vi "A320飞行姿态模拟.vi"() -> ()   [LabVIEW 2014]
uses:
  <vilib>/picture/3D Picture Control/Object/Create Object (name).vi
  <vilib>/picture/3D Picture Control/Object/Add Object (reference).vi
  <vilib>/picture/3D Picture Control/NI_3D Picture Control.lvlib
panel:
  in  "退出按钮":bool
  in  "Yaw":dbl(knob) scale=-180.0..180.0
  in  "Roll":dbl(knob) scale=-90.0..90.0
  in  "Pitch":dbl(knob) scale=-180.0..180.0
  out "三维图片":refnum<vi>(3d-picture)
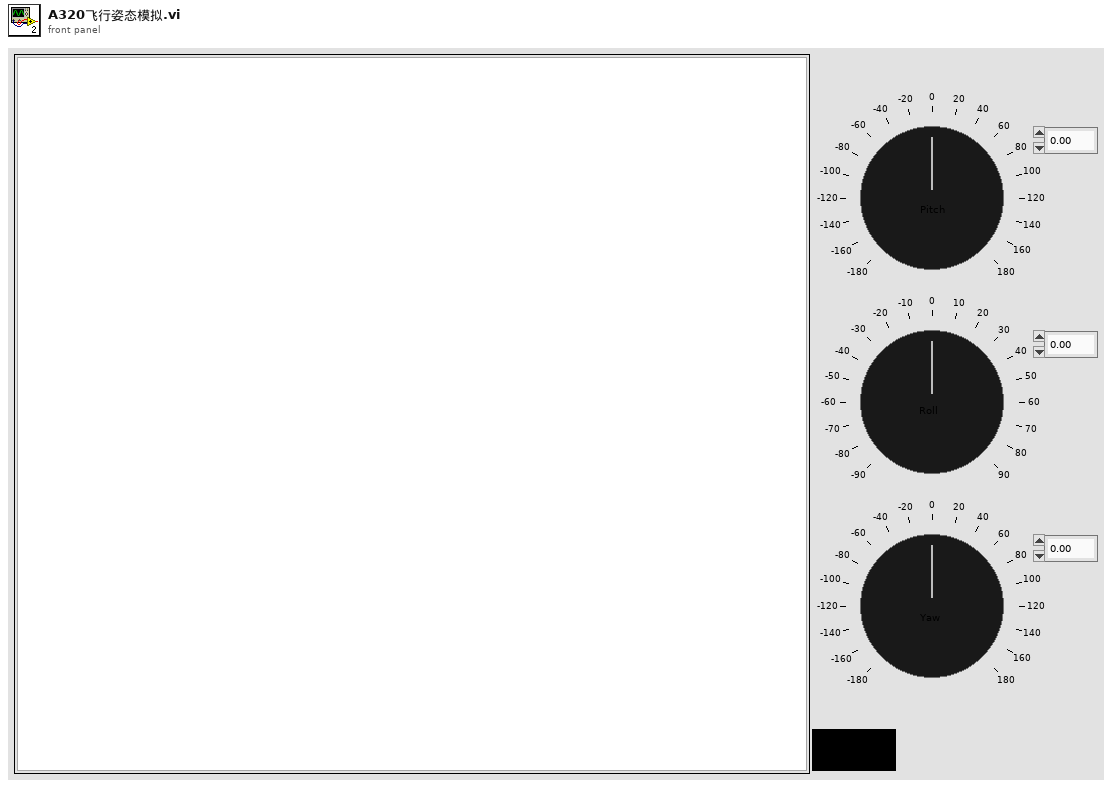
[diagram p1: front panel]
types:
  T1 = cluster{"Red":sgl, "Green":sgl, "Blue":sgl, "Alpha":sgl}
  T2 = enum8{"Enabled", "Disabled", "Disabled and Grayed Out"}
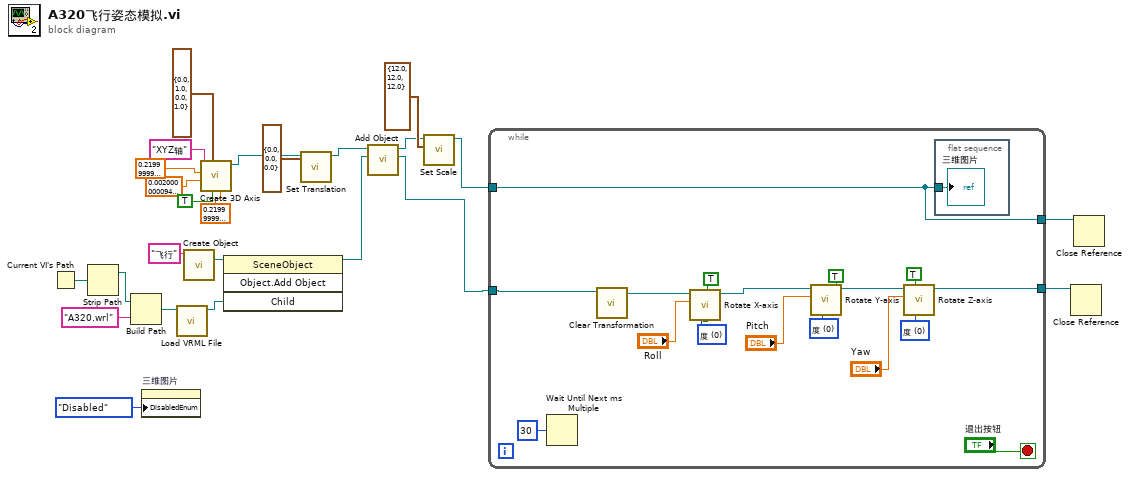
[diagram p0: block diagram]
diagram:
  n1 = Current VI's Path() -> (path=w22:path)
  n2 = Strip Path ("拆分路径")(path=w22) -> (stripped path=w21:path)  [unwired: 1 out]
  n3 = Build Path ("创建路径")(base path=w21, name or relative path="A320.wrl" ("名称或相对路径")) -> (appended path=w19:path)
  n4 = property on="三维图片" class="SceneGraphDisp (严格)"("DisabledEnum"=T2."Disabled" ("禁用")) -> ()  [unwired: 2 in, 2 out]
  n5 = call <vilib>:"Load VRML File.vi"("Path"=w19) -> ("Scene:Read Scene File"=w15:refnum<vi>)  [unwired: 9 in, 1 out]
  n6 = call-poly <vilib>:"Create Object.vi"("Name"="飞行") -> ("Scene:New Object"=w18:refnum<vi>)  [unwired: 9 in, 1 out]
  n7 = call <vilib>:"Create 3D Axis.vi"("Character Size"=sgl 0.22, "Axis label?"=TRUE, "Color"=T1 {"Red"=0.0, "Green"=1.0, "Blue"=0.0, "Alpha"=1.0}, "Radius"=sgl 0.002, "Length"=sgl 0.22, "Name"="XYZ轴") -> ("New Object Refnum"=w7:refnum<vi>)  [unwired: 4 in, 1 out]
  n8 = invoke class="SceneObject" method="Object.Add Object"(reference=w18, "Child"=w15) -> (reference out=w1:refnum<vi>)  [unwired: 2 in, 3 out]
  n9 = call <vilib>:"Set Translation.vi"("Translation"=cluster{"X":sgl, "Y":sgl, "Z":sgl} {"X"=0.0, "Y"=0.0, "Z"=0.0}, "Scene Object"=w7) -> ("Translated Object"=w2:refnum<vi>)  [unwired: 8 in, 1 out]
  n10 = call-poly <vilib>:"Add Object.vi"("New Object In"=w1, "Scene Object In"=w2) -> ("New Object Out"=w3:refnum<vi>, "Scene Object Out"=w8:refnum<vi>)  [unwired: 7 in, 1 out]
  n11 = call <vilib>:"Set Scale.vi"("Scale"=cluster{"X":sgl, "Y":sgl, "Z":sgl} {"X"=12.0, "Y"=12.0, "Z"=12.0}, "Scene Object"=w8) -> ("Scaled Object"=w4:refnum<vi>)  [unwired: 8 in, 1 out]
  n12 = while {
    tunnel: w4 -> [w34]
    tunnel: w3 -> [w25]
    tunnel: [w34] -> w24
    tunnel: [w33] -> w23
    stop <- "退出按钮" stop-if-true
    w39 = u16 0 items=["度", "弧度"] ("angle unit")
    w40 = u16 0 items=["度", "弧度"] ("angle unit")
    w41 = u16 0 items=["度", "弧度"] ("angle unit")
    n13 = Wait Until Next ms Multiple(millisecond multiple=u32 30 ("毫秒倍数")) -> ()  [unwired: 1 out]
    n14 = call <vilib>:"Clear Transformation.vi"("Object Refnum In"=w25) -> ("Object Refnum Out"=w36:refnum<vi>)  [unwired: 9 in, 1 out]
    n15 = call <vilib>:"Rotate X-axis.vi"("angle unit"=w41, "Relative?"=TRUE, "angle"="Roll", "Scene Object In"=w36) -> ("Scene Object Out"=w38:refnum<vi>)  [unwired: 6 in, 1 out]
    n16 = call <vilib>:"Rotate Y-axis.vi"("angle unit"=w40, "Relative?"=TRUE, "angle"="Pitch", "Scene Object In"=w38) -> ("Scene Object Out"=w37:refnum<vi>)  [unwired: 6 in, 1 out]
    n17 = call <vilib>:"Rotate Z-axis.vi"("angle unit"=w39, "Relative?"=TRUE, "angle"="Yaw", "Scene Object In"=w37) -> ("Scene Object Out"=w33:refnum<vi>)  [unwired: 6 in, 1 out]
    n18 = flat-sequence {
      tunnel: w34 -> [w42]
      frame #0 {
        "三维图片" <- w42
      }
    }
  }
  n19 = Close Reference(reference=w23) -> ()  [unwired: 1 in, 1 out]
  n20 = Close Reference(reference=w24) -> ()  [unwired: 1 in, 1 out]
